vi "Create Input Param Route.vi"(10 "Control Terminal":refnum<vi>, 11 "Abstract Param Writer in":refnum<class "Abstract Param Writer.lvclass">) -> (2 "CLFN Terminal Source":refnum<vi>, 3 "Abstract Param Writer out":refnum<class "Abstract Param Writer.lvclass">)   [LabVIEW 2013, in "Abstract Param Writer.lvclass"]
doc: "Subclasses should reimplement this VI to create a route between the control terminal and the CLFN terminal, and add any intermediate nodes required.\n\nThe default implementation simply links the control terminal directly to the CLFN terminal."
uses:
  Abstract Param Writer.lvclass
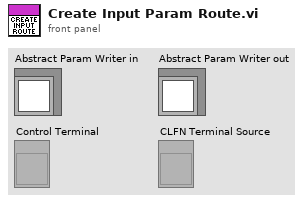
[diagram p1: front panel]
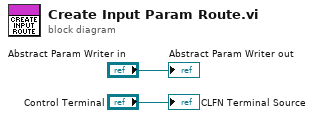
[diagram p0: block diagram]
diagram:
  "Abstract Param Writer out" <- "Abstract Param Writer in"
  "CLFN Terminal Source" <- "Control Terminal"
